vi "CameraStateController.vi"(1 "Selected State (In)":string) -> (0 "Selected State (Out)":string)   [LabVIEW 2019]
uses:
  dsdata.vi
  outputs.vi
  dsinstructions.vi
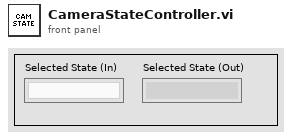
[diagram p1: front panel]
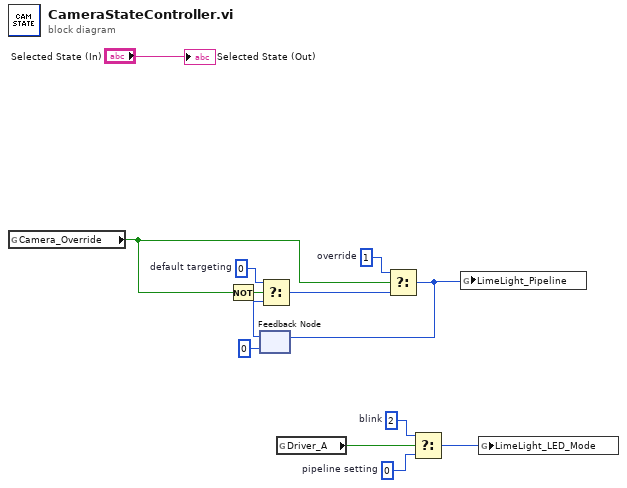
[diagram p0: block diagram]
diagram:
  w2 = i64 0  # pipeline setting
  w4 = i64 2  # blink
  w8 = i64 0  # default targeting
  w9 = i64 1  # override
  n1 = global read "dsdata.vi" "Camera_Override"() -> (w6:bool)
  n2 = Not(x=w6) -> (.not. x?=w7:bool)
  n3 = feedback #1(i64 0 ("t")) -> (w12:i64)
  n4 = Select(t=w8, s=w7, f=w12) -> (s? t:f=w10:i64)
  n5 = global read "dsinstructions.vi" "Driver_A"() -> (w1:bool)
  n6 = Select(t=w9, s=w6, f=w10) -> (s? t:f=w5:i64)
  n7 = feedback-in #1(w5) -> ()
  n8 = Select(t=w4, s=w1, f=w2) -> (s? t:f=w3:i64)
  n9 = global write "outputs.vi" "LimeLight_Pipeline"(w5) -> ()
  n10 = global write "outputs.vi" "LimeLight_LED_Mode"(w3) -> ()
  "Selected State (Out)" <- "Selected State (In)"
